vi "Testing.vi"() -> ()   [LabVIEW 2015]
uses:
  <vilib>/Utility/file.llb/Read Delimited Spreadsheet (string).vi
panel:
  out "Start Y":dbl
  out "Start X":dbl
  out "Starting Point":string
  out "Table":string[][](table)
  in  "Centers":path
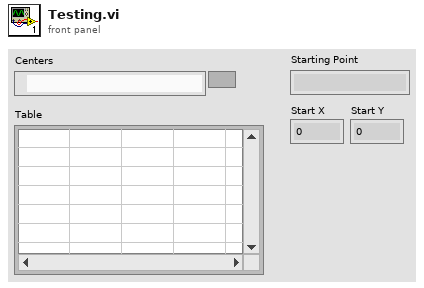
[diagram p1: front panel]
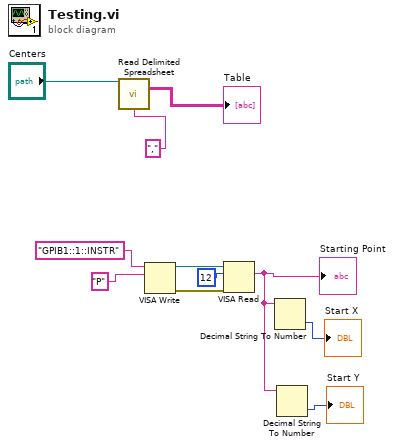
[diagram p0: block diagram]
diagram:
  n1 = call-poly <vilib>:"Read Delimited Spreadsheet.vi"("file path (dialog if empty)"="Centers", "delimiter (\\t)"=",") -> ("all rows"=→"Table":string[][])  [unwired: 8 in, 5 out]
  n2 = VISA Write(VISA resource name="GPIB1::1::INSTR", write buffer="P") -> (VISA resource name out=w6:refnum<visa-resource-name>, error out=w5:errorcluster)  [unwired: 1 in, 1 out]
  n3 = VISA Read(VISA resource name=w6, byte count=12, error in (no error)=w5) -> (read buffer=w1:string)  [unwired: 3 out]
  "Starting Point" <- w1
  n4 = Decimal String To Number(string=w1) -> (number=→"Start X":i32)  [unwired: 2 in, 1 out]
  n5 = Decimal String To Number(string=w1) -> (number=→"Start Y":i32)  [unwired: 2 in, 1 out]
